vi "Intake Control.vi"(8 "Forward/Reverse":bool, 10 "Enum":T1) -> ()   [LabVIEW 2014]
uses:
  SRE Enum.ctl
  <vilib>/Rock Robotics/WPI/Solenoid/WPI_SolenoidValue.ctl
  <vilib>/Rock Robotics/WPI/Solenoid/WPI_SolenoidOpenDouble.vi
  <vilib>/Rock Robotics/WPI/Solenoid/WPI_SolenoidSetEnum.vi
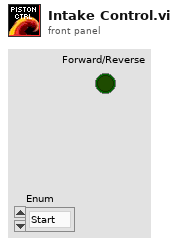
[diagram p1: front panel]
types:
  T1 = typedef "SRE Enum.ctl" = enum16{"Start", "Run", "End"}
  T2 = typedef "WPI_SolenoidValue.ctl" = enum16{"Off", "On", "Forward", "Reverse"}
  T3 = typedef "WPI_SolenoidDevRef.ctl" = cluster{"DevStatus":errorcluster, "Pneumatics Control Module":u8, "Forward Solenoid Channel":T4, "Reverse Solenoid Channel":T4}
  T4 = typedef "WPI_SolenoidChannel.ctl" = enum8{"Solenoid 0", "Solenoid 1", "Solenoid 2", "Solenoid 3", "Solenoid 4", "Solenoid 5", "Solenoid 6", "Solenoid 7", "Invalid"}
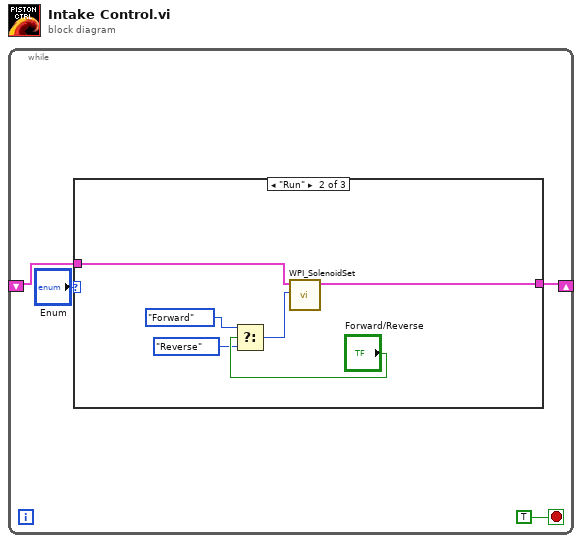
[diagram p0: block diagram]
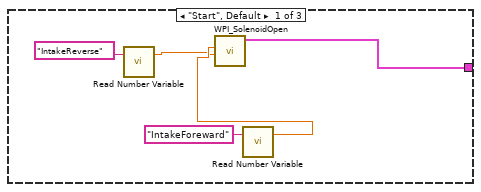
[diagram p2: hidden frame]
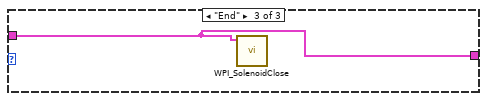
[diagram p3: hidden frame]
diagram:
  n1 = while {
    shift-right: [w3] -> _
    shift-left: _ -> [w2]
    stop <- TRUE stop-if-true
    n2 = case shown="\"Run\"" "Enum" {
      tunnel: [w9 w15 w16] -> w3
      tunnel: w2 -> [_ w14 w16]
      frame "Start", Default {
        n3 = call "Read Number Variable.vi"("Name"="IntakeReverse") -> ("number"=w5:dbl)  [unwired: 1 in, 1 out]
        n4 = call "Read Number Variable.vi"("Name"="IntakeForeward") -> ("number"=w7:dbl)  [unwired: 1 in, 1 out]
        n5 = call-poly <vilib>:"WPI_SolenoidOpen.vi"("Reverse Solenoid Channel"=w5, "Forward Solenoid Channel"=w7) -> ("SolenoidDevRef"=w9:T3)  [unwired: 8 in, 1 out]
      }
      frame "Run" {
        n6 = Select(t=WPI_SolenoidValue."Forward" ("Value"), s="Forward/Reverse", f=WPI_SolenoidValue."Reverse") -> (s? t:f=w11:T2)
        n7 = call-poly <vilib>:"WPI_SolenoidSet.vi"("Value"=w11, "SolenoidDevRef"=w14) -> ("SolenoidDevRef"=w15:T3)  [unwired: 8 in, 1 out]
      }
      frame "End" {
        n8 = call <vilib>:"WPI_SolenoidClose.vi"("SolenoidDevRef"=w16) -> ()  [unwired: 10 in, 1 out]
      }
    }
  }
